vi "Measure Digital Signal.vi"(0 "Data In":bool) -> (4 "Data Out":bool, 6 "F-F Delta (Ticks)":u32, 8 "F-R Delta(Ticks)":u32, 10 "R-R Delta (Ticks)":u32, 15 "R-F Delta (Ticks)":u32)   [LabVIEW 2024]
doc: "Measures the rising edge to falling edge delta in ticks of the FPGA clock."
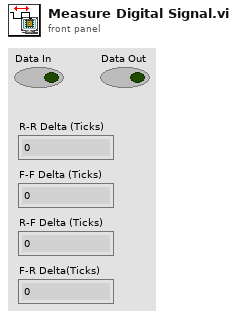
[diagram p1: front panel]
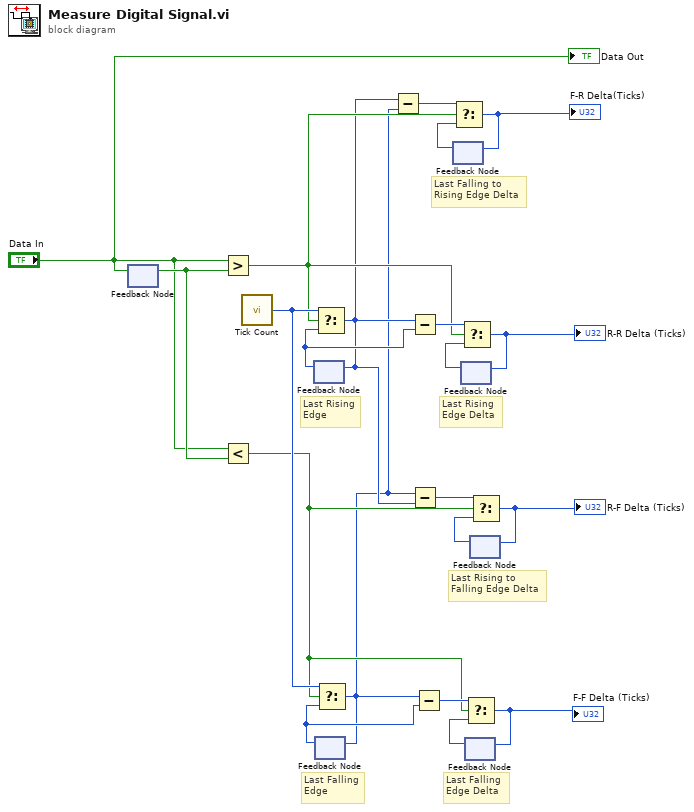
[diagram p0: block diagram]
diagram:
  # "Last Falling to\nRising Edge Delta"
  # "Last Falling \nEdge Delta"
  # "Last Rising to\nFalling Edge Delta"
  # "Last Falling\nEdge"
  # "Last Rising \nEdge Delta"
  # "Last Rising\nEdge"
  n1 = feedback #1() -> (w13:bool)  [unwired: 1 in]
  n2 = feedback-in #1("Data In") -> ()
  n3 = Greater?(x="Data In", y=w13) -> (0:w3:bool)
  n4 = Less?(x="Data In", y=w13) -> (x < y?=w8:bool)
  n5 = call "Tick Count"() -> ("Tick Count(Ticks)"=w18:u32)
  n6 = feedback #2() -> (w14:u32)  [unwired: 1 in]
  n7 = feedback #3() -> (w7:u32)  [unwired: 1 in]
  n8 = Select(t=w18, s=w3, f=w14) -> (s? t:f=w2:u32)
  n9 = feedback-in #2(w2) -> ()
  n10 = Select(t=w18, s=w8, f=w7) -> (s? t:f=w1:u32)
  n11 = feedback-in #3(w1) -> ()
  n12 = Subtract(x=w2, y=w1) -> (x-y=w6:u32)
  n13 = Subtract(x=w2, y=w14) -> (x-y=w15:u32)
  n14 = Subtract(x=w1, y=w2) -> (x-y=w21:u32)
  n15 = Subtract(x=w1, y=w7) -> (x-y=w9:u32)
  n16 = feedback #4() -> (w5:u32)  [unwired: 1 in]
  n17 = Select(t=w6, s=w3, f=w5) -> (s? t:f=w4:u32)
  "F-R Delta(Ticks)" <- w4
  n18 = feedback-in #4(w4) -> ()
  n19 = feedback #5() -> (w17:u32)  [unwired: 1 in]
  n20 = Select(t=w15, s=w3, f=w17) -> (s? t:f=w16:u32)
  "R-R Delta (Ticks)" <- w16
  n21 = feedback-in #5(w16) -> ()
  n22 = feedback #6() -> (w11:u32)  [unwired: 1 in]
  n23 = Select(t=w9, s=w8, f=w11) -> (s? t:f=w10:u32)
  "F-F Delta (Ticks)" <- w10
  n24 = feedback-in #6(w10) -> ()
  n25 = feedback #7() -> (w20:u32)  [unwired: 1 in]
  n26 = Select(t=w21, s=w8, f=w20) -> (s? t:f=w19:u32)
  "R-F Delta (Ticks)" <- w19
  n27 = feedback-in #7(w19) -> ()
  "Data Out" <- "Data In"
